vi "Test Tab Control Ref.vi"(7 "Page Label":string="Page 1", 8 "error in":errorcluster, 11 "TabControl Reference":refnum<vi>) -> (0 "error out":errorcluster, 2 "Array Out":string[](array[string]), 3 "Array":refnum<vi>[](array[refnum]))   [LabVIEW 2022 SP3]
panel:
  in  "Tab Control":enum32{"Page 1", "Page 2"}(tab)
  out "Boolean 2":bool
  out "Boolean":bool
  out "Array 3":string[](array[string])
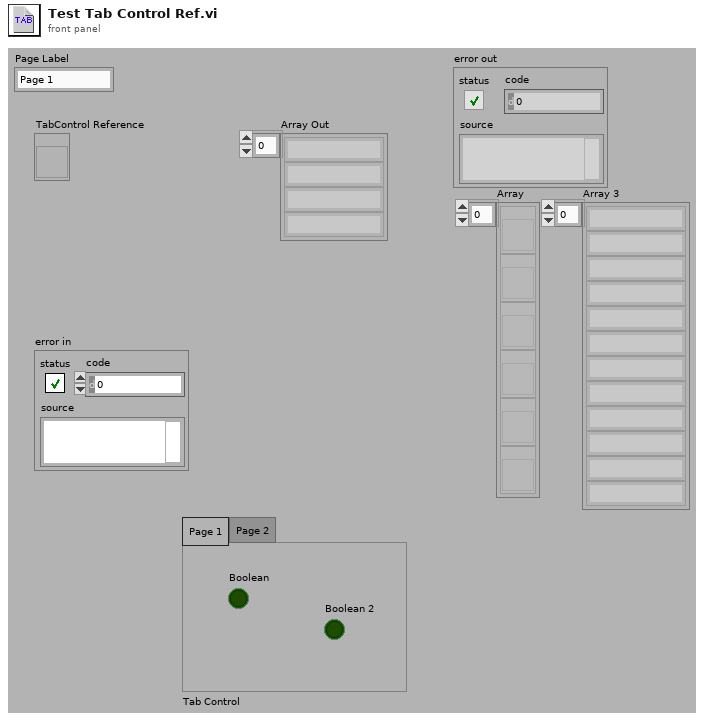
[diagram p1: front panel]
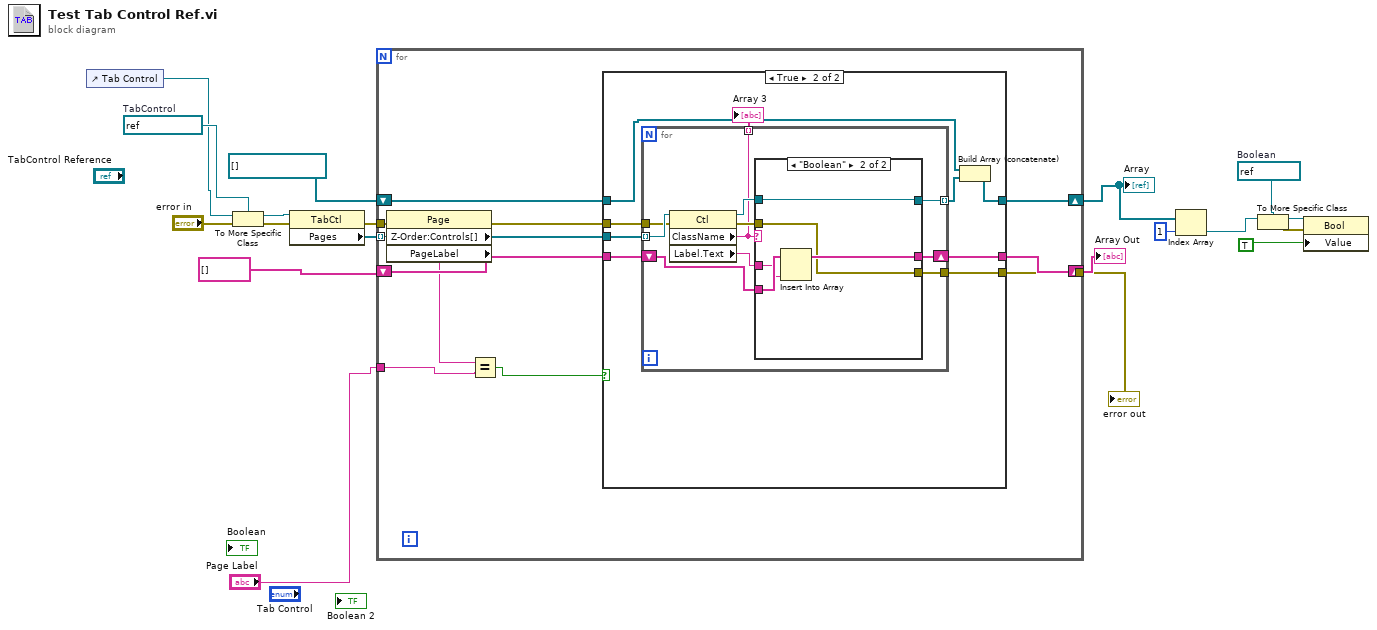
[diagram p0: block diagram]
diagram:
  w5 = refnum<vi> refnum  # Boolean
  w16 = refnum<vi> refnum  # TabControl
  n1 = control-ref of="Tab Control"() -> (w8:refnum<vi>)
  n2 = To More Specific Class(target class=w16, reference=w8, error in="error in") -> (specific class reference=w14:refnum<vi>, error out=w13:errorcluster)
  n3 = property class="TabCtl"(reference=w14, error in=w13) -> (error out=w19:errorcluster, "Pages"=w17:refnum<vi>[])  [unwired: 1 out]
  n4 = for {
    tunnel: w17 -> [w31] mode=indexing
    shift-right: [w29] -> w18
    shift-left: string[] [] ("Array In") -> [w28]
    tunnel: w19 -> [w27]
    tunnel: "Page Label" -> [w24]
    tunnel: [w22] -> w11
    shift-right: [w21] -> w7
    shift-left: refnum<vi>[] [] ("Array 2") -> [w20]
    n5 = property class="Page"(reference=w31, error in=w27) -> (error out=w26:errorcluster, "Z-Order:Controls[]"=w30:refnum<vi>[], "PageLabel"=w25:string)  [unwired: 1 out]
    n6 = Equal?(x=w25, y=w24) -> (x = y?=w23:bool)
    n7 = case shown="True" w23 {
      tunnel: w30 -> [_ w43]
      tunnel: [w34 w42] -> w29
      tunnel: w28 -> [w34 w41]
      tunnel: w26 -> [w33 w40]
      tunnel: [w33 w39] -> w22
      tunnel: [w32 w36] -> w21
      tunnel: w20 -> [w32 w38]
      frame False {
      }
      frame True {
        n8 = for {
          tunnel: w43 -> [w51] mode=indexing
          shift-right: [w52] -> w42
          shift-left: w41 -> [w53]
          tunnel: w40 -> [w50]
          tunnel: [w46] -> w39
          tunnel: [w45] -> w37 mode=indexing
          tunnel: [w44] -> w35 mode=indexing
          n9 = property class="Ctl"(reference=w51, error in=w50) -> (reference out=w48:refnum<vi>, error out=w47:errorcluster, "ClassName"=w44:string, "Label.Text"=w49:string)
          n10 = case shown="\"Boolean\"" w44 {
            tunnel: w53 -> [w54 w61]
            tunnel: [w54 w59] -> w52
            tunnel: w49 -> [_ w60]
            tunnel: w48 -> [w55 w57]
            tunnel: w47 -> [w56 w58]
            tunnel: [w56 w58] -> w46
            tunnel: [w55 w57] -> w45
            frame "", Default {
            }
            frame "Boolean" {
              n11 = Insert Into Array(array=w61, new element=w60) -> (w59:string[])  [unwired: 1 in]
            }
          }
        }
        "Array 3" <- w35
        n12 = Build Array (concatenate)(w38, w37) -> (w36:refnum<vi>[])
      }
    }
  }
  "Array Out" <- w18
  "error out" <- w11
  "Array" <- w7
  n13 = Index Array(array=w7, index=1) -> (element=w2:refnum<vi>)
  n14 = To More Specific Class(target class=w5, reference=w2) -> (specific class reference=w4:refnum<vi>, error out=w3:errorcluster)  [unwired: 1 in]
  n15 = property class="Bool"(reference=w4, error in=w3, "Value"=TRUE) -> ()  [unwired: 2 out]
